vi "extract exifinfo.vi"(8 "error in":errorcluster, 11 "file path":path) -> (0 "error out":errorcluster, 2 "Array":string[][](array[string]), 3 "Info":T1={"Make"="Canon\u0000", "Model"="Canon PowerShot A495\u0000", "Orientation"=0, "Date"=timestamp(0 s since 1904-01-01), "Width"=0, "Height"=0, "Square?"=FALSE, "File Name"="Canon\u0000", "Extension"="Canon\u0000", "Valid?"=FALSE, "Path"=path "", "size"=0, "No Ext?"=FALSE, "prefix?"=FALSE, "String"="", "Name Type"=enum."Event Sufix"})   [LabVIEW 2023, in "File Classes.lvlib" / "Picture File.lvclass"]
uses:
  Picture File.lvclass
  Controls/exif data cluster.ctl
  Controls/rename type enum.ctl
  File Classes.lvlib
panel:
  # "D:\\Library\\Pictures\\Photos\\Pollachi iPhone Videos\\2024-12-24 003.MOV"
  # "D:\\Library\\Pictures\\Photos\\Pollachi Nikon 5600 Videos\\DSC_0229.MOV"
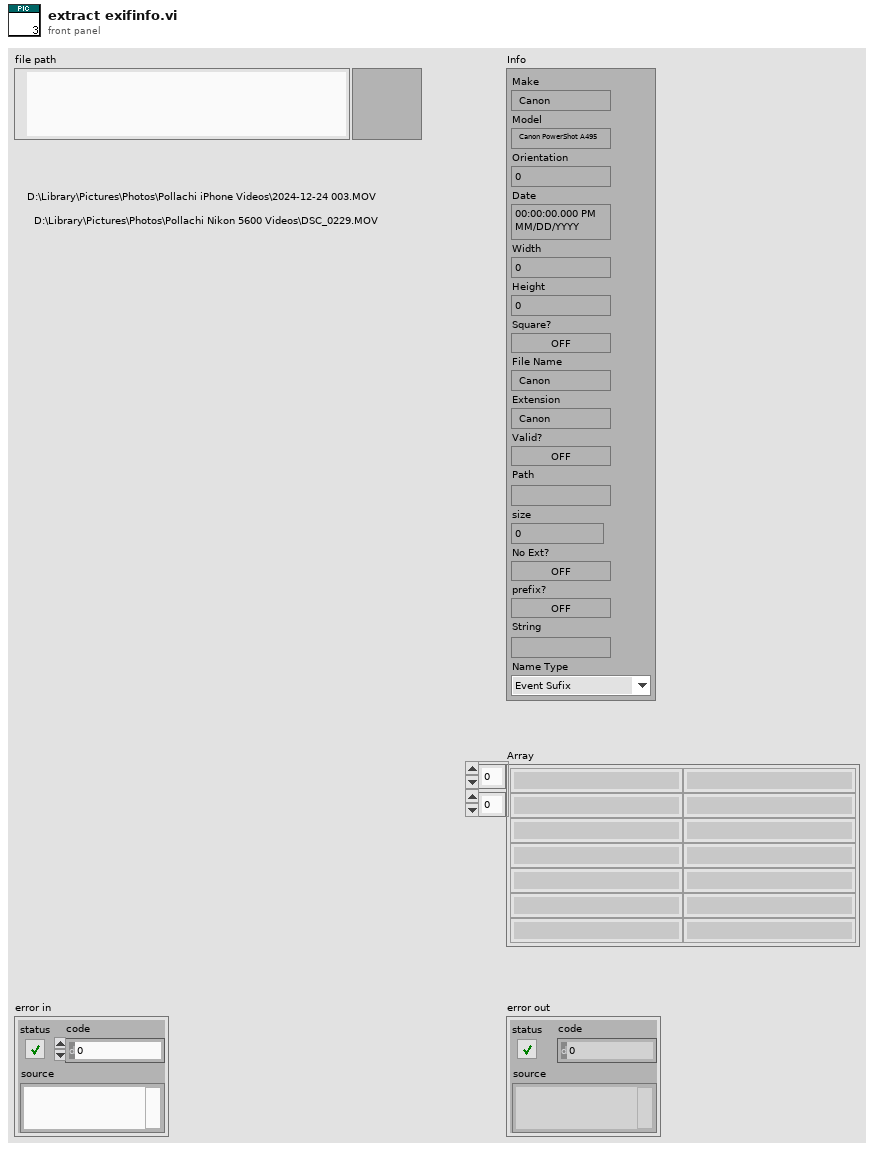
[diagram p1: front panel]
types:
  T1 = typedef "File Classes.lvlib/exif data cluster.ctl" = cluster{"Make":string, "Model":string, "Orientation":u16, "Date":timestamp, "Width":u16, "Height":u16, "Square?":bool, "File Name":string, "Extension":string, "Valid?":bool, "Path":path, "size":i64, "No Ext?":bool, "prefix?":bool, "String":string, "Name Type":T2}
  T2 = typedef "File Classes.lvlib/rename type enum.ctl" = enum16{"Date & Time (Default)", "Model Sufix", "Event Sufix", "Model & Event Sufix"}
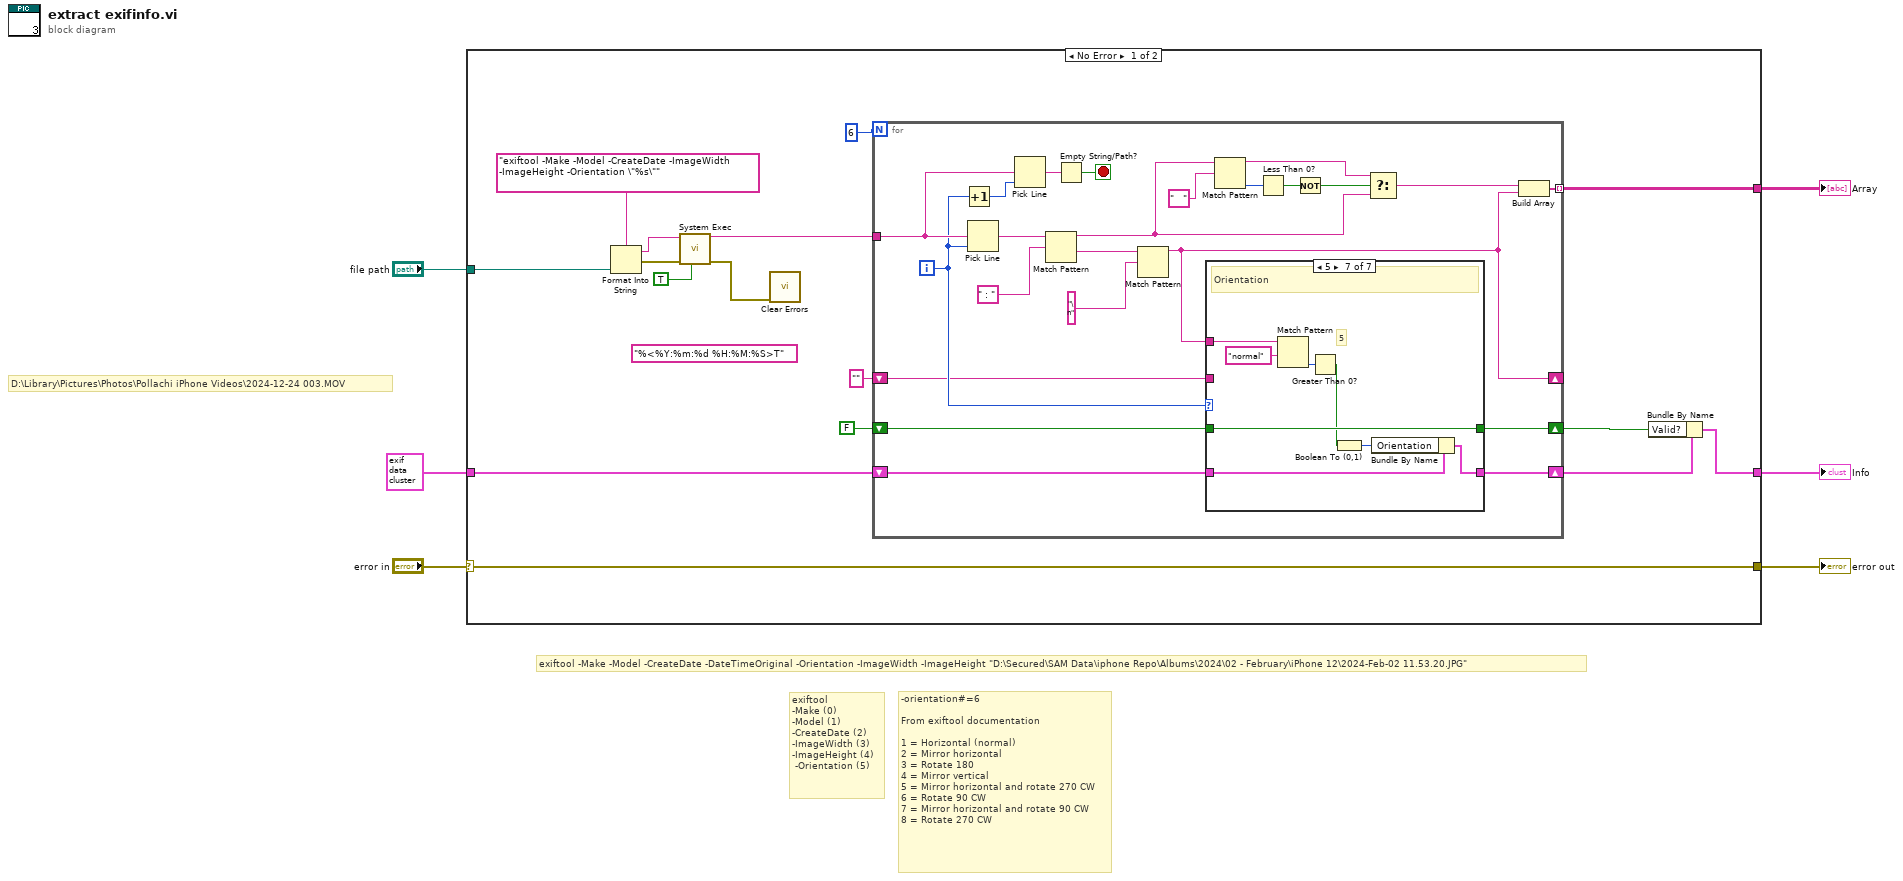
[diagram p0: block diagram]
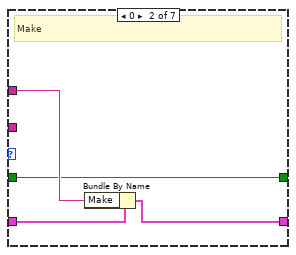
[diagram p3: hidden frame]
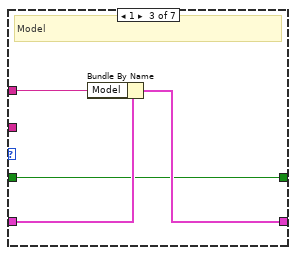
[diagram p4: hidden frame]
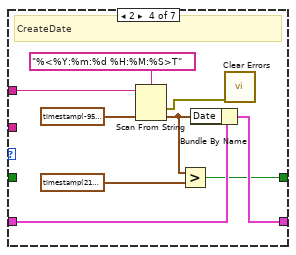
[diagram p5: hidden frame]
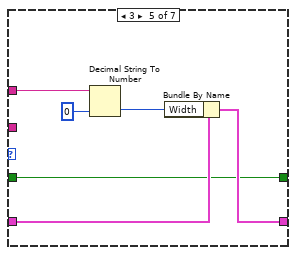
[diagram p6: hidden frame]
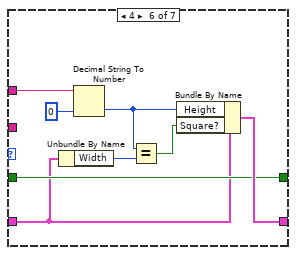
[diagram p7: hidden frame]
diagram:
  # "D:\\Library\\Pictures\\Photos\\Pollachi iPhone Videos\\2024-12-24 003.MOV"
  # "-orientation#=6\n\nFrom exiftool documentation\n\n1 = Horizontal (normal)\n2 = Mirror horizontal\n3 = Rotate 180\n4 = Mirror vertical\n5 = Mirror horizontal and rotate 270 CW\n6 = Rotate 90 CW\n7 = Mirror horizontal and rotate 90 CW\n8 = Rotate 270 CW"
  # "exiftool -Make -Model -CreateDate -DateTimeOriginal -Orientation -ImageWidth -ImageHeight \"D:\\Secured\\SAM Data\\iphone Repo\\Albums\\2024\\02 - February\\iPhone 12\\2024-Feb-02 11.53.20.JPG\""
  # "exiftool \n-Make (0) \n-Model (1)\n-CreateDate (2) \n-ImageWidth (3)\n-ImageHeight (4)\n -Orientation (5)"
  n1 = case shown="No Error" "error in" {
    selector: "error in" -> [w13 w88]
    tunnel: "file path" -> [w18 _]
    tunnel: [w17 _] -> w5
    tunnel: [w10 w87] -> w4
    tunnel: [w13 w88] -> w2
    tunnel: T1 {"Make"="Make", "Model"="model", "Orientation"=0, "Date"=timestamp(3799139022 s since 1904-01-01), "Width"=3, "Height"=4, "Square?"=FALSE, "File Name"="Canon\u0000", "Extension"="Canon\u0000", "Valid?"=FALSE, "Path"=path "", "size"=0, "No Ext?"=FALSE, "prefix?"=FALSE, "String"="", "Name Type"=enum."Date & Time (Default)"} ("Info") -> [w11 w87]
    frame No Error {
      (unwired) "%<%Y:%m:%d %H:%M:%S>T" ("format string")
      n2 = Format Into String(format string="exiftool -Make -Model -CreateDate -ImageWidth -ImageHeight -Orientation \"%s\"" ("command line"), w18) -> (resulting string=w20:string, error out=w19:errorcluster)  [unwired: 2 in]
      n3 = call <vilib>:"System Exec.vi"("run minimized? (F)"=TRUE, "error in (no error)"=w19, "command line"=w20) -> ("error out"=w12:errorcluster, "standard output"=w15:string)  [unwired: 5 in, 2 out]
      n4 = call <vilib>:"Clear Errors.vi"("error in (no error)"=w12) -> ()  [unwired: 5 in, 2 out]
      n5 = for {
        N: 6 -> [_]
        tunnel: w15 -> [w34]
        tunnel: [w36] -> w17 mode=indexing
        shift-right: [w27] -> _
        shift-left: "" ("output string") -> [w28]
        shift-right: [w25] -> w8
        shift-left: FALSE -> [w26]
        shift-right: [w24] -> w14
        shift-left: w11 -> [w23]
        i -> [w29]
        stop <- w30 stop-if-true
        n6 = Increment(x=w29) -> (x+1=w33:i32)
        n7 = Pick Line(multi-line string=w34, line index=w29) -> (output string=w43:string)  [unwired: 1 in]
        n8 = Pick Line(multi-line string=w34, line index=w33) -> (output string=w32:string)  [unwired: 1 in]
        n9 = Match Pattern(string=w43, regular expression=" : ") -> (before substring=w39:string, after substring=w44:string)  [unwired: 1 in, 2 out]
        n10 = Empty String/Path?(string/path=w32) -> (empty?=w30:bool)
        n11 = Match Pattern(string=w44, regular expression="\n") -> (before substring=w27:string)  [unwired: 1 in, 3 out]
        n12 = case shown="5" w29 {
          tunnel: w28 -> [_ _ _ _ _ _ _]
          tunnel: w27 -> [_ w49 w53 w62 w67 w76 w79]
          tunnel: w26 -> [w47 w48 w52 _ w68 w77 w84]
          tunnel: [w47 w48 w52 w58 w68 w77 w84] -> w25
          tunnel: [w46 w50 w54 w63 w69 w78 w85] -> w24
          tunnel: w23 -> [w46 w51 w55 w64 w70 w74 w86]
          frame Default {
          }
          frame 0 {
            # "Make"
            n13 = Bundle By Name(cluster=w51, "Make"=w49) -> (w50:T1)
          }
          frame 1 {
            # "Model"
            n14 = Bundle By Name(cluster=w55, "Model"=w53) -> (w54:T1)
          }
          frame 2 {
            # "CreateDate"
            n15 = Scan From String(format string="%<%Y:%m:%d %H:%M:%S>T", input string=w62, default 1=timestamp(-9568800000 s since 1904-01-01)) -> (error out=w61:errorcluster, output 1=w57:timestamp)  [unwired: 2 in, 2 out]
            n16 = Greater?(x=w57, y=timestamp(2107209600 s since 1904-01-01)) -> (0:w58:bool)
            n17 = Bundle By Name(cluster=w64, "Date"=w57) -> (w63:T1)
            n18 = call <vilib>:"Clear Errors.vi"("error in (no error)"=w61) -> ()  [unwired: 5 in, 2 out]
          }
          frame 3 {
            n19 = Decimal String To Number(string=w67, default (0L)=u16 0 ("Width")) -> (number=w66:u16)  [unwired: 1 in, 1 out]
            n20 = Bundle By Name(cluster=w70, "Width"=w66) -> (w69:T1)
          }
          frame 4 {
            n21 = Unbundle By Name(w74) -> ("Width"=w71:u16)
            n22 = Decimal String To Number(string=w76, default (0L)=u16 0 ("Width")) -> (number=w72:u16)  [unwired: 1 in, 1 out]
            n23 = Equal?(x=w72, y=w71) -> (x = y?=w73:bool)
            n24 = Bundle By Name(cluster=w74, "Height"=w72, "Square?"=w73) -> (w78:T1)
          }
          frame 5 {
            # "5"
            # "Orientation"
            n25 = Match Pattern(string=w79, regular expression="normal") -> (offset past match=w82:i32)  [unwired: 1 in, 3 out]
            n26 = Greater Than 0?(x=w82) -> (x > 0?=w81:bool)
            n27 = Boolean To (0,1)(Boolean=w81) -> (0, 1=w80:i16)
            n28 = Bundle By Name(cluster=w86, "Orientation"=w80) -> (w85:T1)
          }
        }
        n29 = Match Pattern(string=w39, regular expression="   ") -> (before substring=w38:string, offset past match=w40:i32)  [unwired: 1 in, 2 out]
        n30 = Less Than 0?(x=w40) -> (x < 0?=w41:bool)
        n31 = Not(x=w41) -> (.not. x?=w35:bool)
        n32 = Select(t=w38, s=w35, f=w39) -> (s? t:f=w37:string)
        n33 = Build Array(w37, w27) -> (w36:string[])
      }
      n34 = Bundle By Name(cluster=w14, "Valid?"=w8) -> (w10:T1)
    }
    frame Error {
    }
  }
  "Array" <- w5
  "Info" <- w4
  "error out" <- w2
